vi "coerce to range.vi"(7 "coerce? (T)":bool=TRUE, 9 "min":dbl, 10 "value in":dbl, 11 "max":dbl) -> (1 "in range":bool, 2 "value out":dbl)   [LabVIEW 2009]
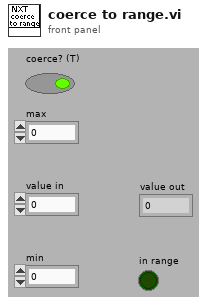
[diagram p1: front panel]
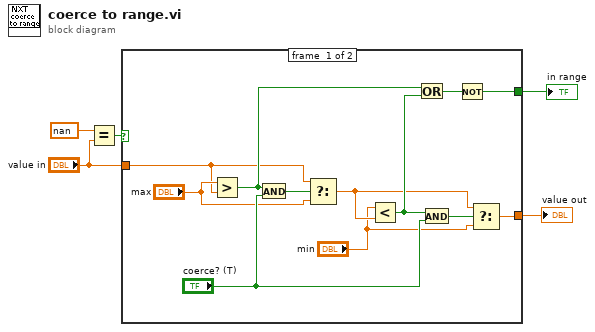
[diagram p0: block diagram]
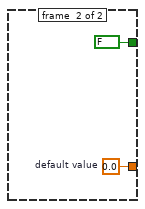
[diagram p2: hidden frame]
diagram:
  n1 = Equal?(x=nan, y="value in") -> (x = y?=w3:bool)
  n2 = case shown="True" w3 {
    tunnel: [w16 w18] -> w5
    tunnel: [w10 FALSE] -> w4
    tunnel: "value in" -> [w6 _]
    frame #0 {
      n3 = Greater?(x="max", y=w6) -> (0:w12:bool)
      n4 = And(x=w12, y="coerce? (T)") -> (x .and. y?=w17:bool)
      n5 = Select(t=w6, s=w17, f="max") -> (s? t:f=w8:dbl)
      n6 = Less?(x="min", y=w8) -> (x < y?=w11:bool)
      n7 = Or(x=w12, y=w11) -> (x .or. y?=w14:bool)
      n8 = And(x=w11, y="coerce? (T)") -> (x .and. y?=w13:bool)
      n9 = Not(x=w14) -> (.not. x?=w10:bool)
      n10 = Select(t=w8, s=w13, f="min") -> (s? t:f=w16:dbl)
    }
    frame #1 {
      w18 = 0.0  # default value
    }
  }
  "value out" <- w5
  "in range" <- w4
